vi "MK210.vi"(4 "error in":T13, 7 "Command":T14) -> (0 "error out":T13, 3 "Response":T11)   [LabVIEW 2018]
uses:
  MOKO_LabViewLibrary/MokoLowLevel/MokoLowLovelControl/MLLC_Command.ctl
  MOKO_LabViewLibrary/MokoLowLevel/MokoLowLovelControl/MLLC_Error.ctl
  MOKO_LabViewLibrary/MokoLowLevel/MokoLowLovelControl/MLLC_Mode.ctl
  MOKO_LabViewLibrary/MokoLowLevel/MokoLowLovelControl/MLLC_Response.ctl
  MOKO_LabViewLibrary/MokoLowLevel/MokoLowLovelControl/MLLC_DriverName.ctl
  MOKO_LabViewLibrary/MokoLowLevel/MokoLowLovelControl/MLLC_ResponseInit.ctl
  MOKO_LabViewLibrary/MokoLowLevel/MokoLowLovelControl/MLLC_Request.ctl
  MOKO_LabViewLibrary/MokoLowLevel/MokoLowLovelControl/MLLC_ErrorCode.ctl
  MOKO_LabViewLibrary/MokoLowLevel/MokoLowLovelControl/MLLC_ConnectCluster.ctl
  MOKO_LabViewLibrary/MokoLowLevel/MokoLowLovelControl/MLLC_InterfaceType.ctl
  MOKO_LabViewLibrary/MokoLowLevel/MokoLowLovelControl/MLLC_OpenedSession.ctl
  MOKO_LabViewLibrary/MokoLowLevel/MokoLowLovelControl/MLLC_InterfaceSettings.ctl
  MOKO_LabViewLibrary/MokoLowLevel/MokoLowLovelControl/MLLC_InterfaceKind.ctl
  MOKO_LabViewLibrary/MokoLowLevel/MokoLowLovelControl/MLLC_Rs232Settings.ctl
panel:
  in  "Settings":T6={"Permanent data"={"Connect"={"InterfaceType"=enum."VISA", "OpenedSession"="COM4", "InterfaceSettings"={"Interface"=enum."RS232", "EOS 4 read"=enum."Default (=EOS 4 write)", "EOS 4 write"=enum."CR (\\r)", "TMO, ms"=500, "Sett"=variant(cluster{"Baud Rate":u32, "Data Bits":u16, "Parity":u16, "Stop Bits":u16, "Flow Control":u16, "Eho":bool} {"Baud Rate"=75, "Data Bits"=0, "Parity"=0, "Stop Bits"=0, "Flow Control"=0, "Eho"=FALSE})}}}, "Saved Data"=variant}
  in  "Error Code":T7=5420
  in  "Request":T8="?MOD"
  in  "ResponseInit":T9="XP2I"
  in  "Driver Name":T10="MK210-301"
  in  "Mode":T12=enum."Check"
  # "MK210-301"
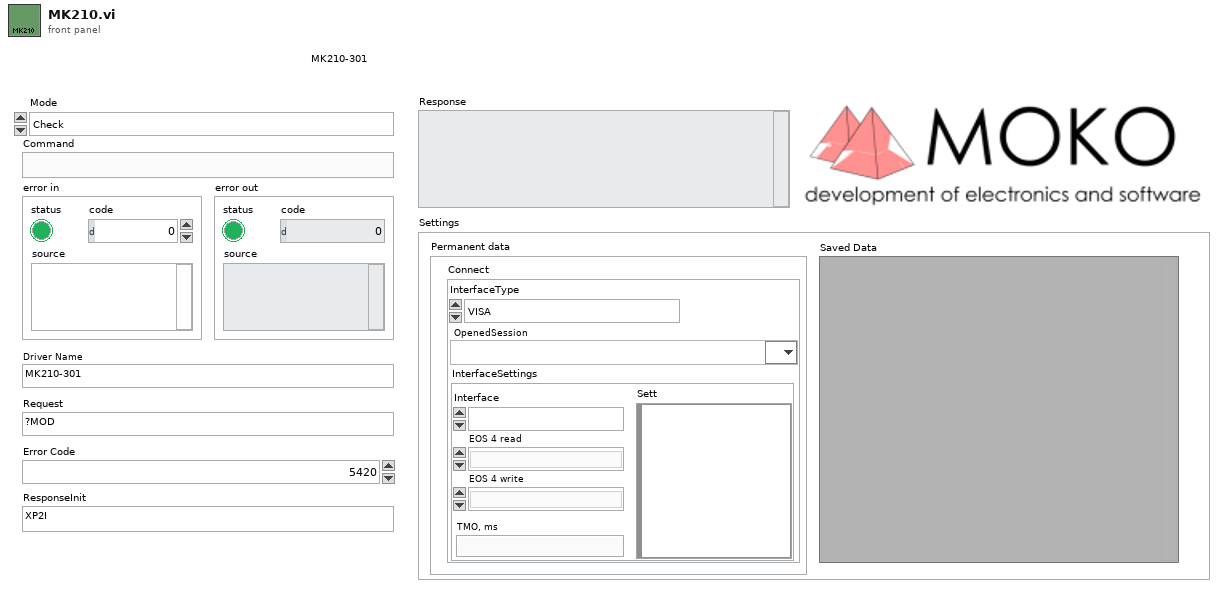
[diagram p1: front panel]
types:
  T1 = typedef "MLLC_ConnectCluster.ctl" = cluster{"InterfaceType":T2, "OpenedSession":T3, "InterfaceSettings":T4}
  T2 = typedef "MLLC_InterfaceType.ctl" = enum16{"VISA", "Prologix USB-GPIB"}
  T3 = typedef "MLLC_OpenedSession.ctl" = refnum<visa-resource-name>
  T4 = typedef "MLLC_InterfaceSettings.ctl" = cluster{"Interface":T5, "EOS 4 read":enum16{"Default (=EOS 4 write)", "CR (\\r)", "LF (\\n)", "None"}, "EOS 4 write":enum16{"CR+LF (\\r\\n)", "CR (\\r)", "LF (\\n)", "None"}, "TMO, ms":i32, "Sett":variant}
  T5 = typedef "MLLC_InterfaceKind.ctl" = enum16{"RS232", "GPIB", "USB", "Ethernet", "another"}
  T6 = cluster{"Permanent data":cluster{"Connect":T1}, "Saved Data":variant}
  T7 = typedef "MLLC_ErrorCode.ctl" = u32
  T8 = typedef "MLLC_Request.ctl" = string
  T9 = typedef "MLLC_ResponseInit.ctl" = string
  T10 = typedef "MLLC_DriverName.ctl" = string
  T11 = typedef "MLLC_Response.ctl" = string
  T12 = typedef "MLLC_Mode.ctl" = enum16{"get", "set", "close", "Init", "Check"}
  T13 = typedef "MLLC_Error.ctl" = errorcluster
  T14 = typedef "MLLC_Command.ctl" = string
  T15 = typedef "MLLC_Rs232Settings.ctl" = cluster{"Baud Rate":u32, "Data Bits":u16, "Parity":u16, "Stop Bits":u16, "Flow Control":u16, "Eho":bool, "Address":dbl}
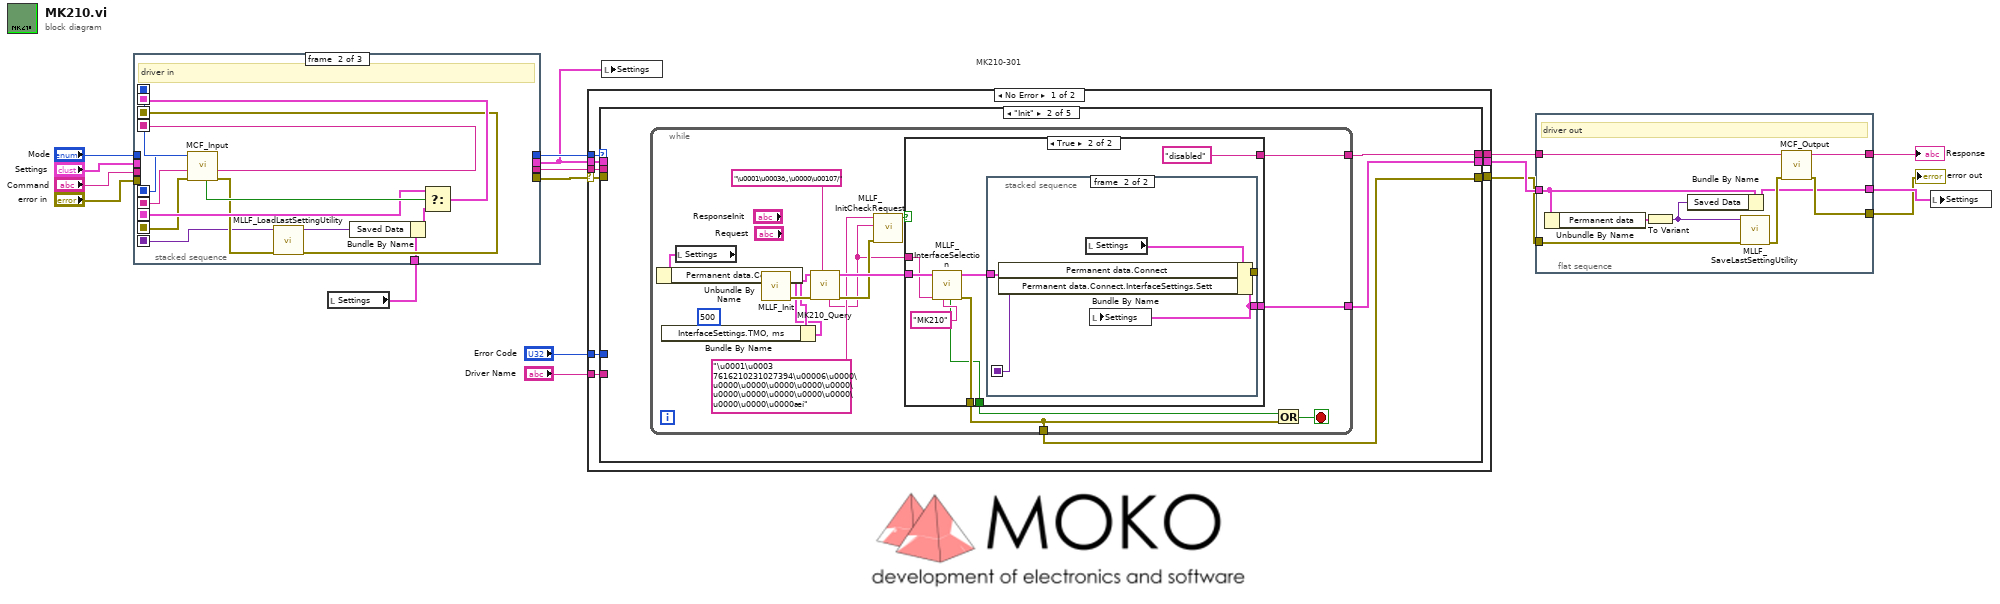
[diagram p0: block diagram]
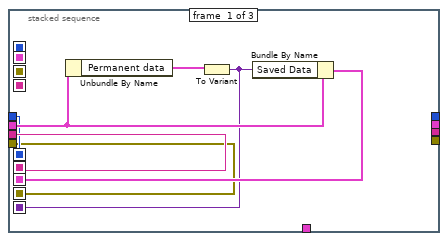
[diagram p2: hidden frame]
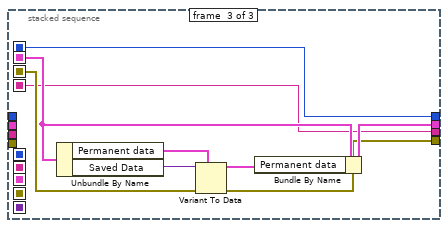
[diagram p3: hidden frame]
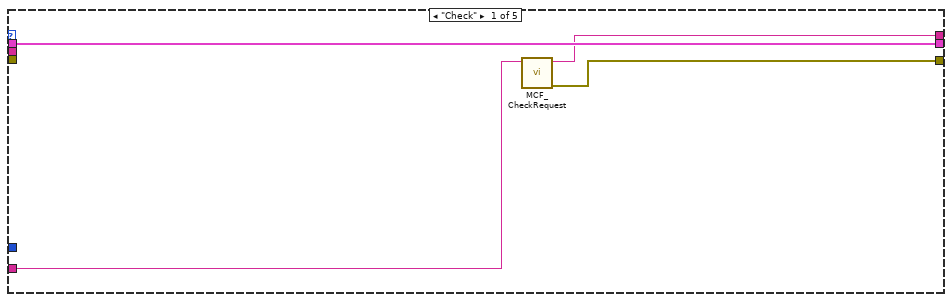
[diagram p4: hidden frame]
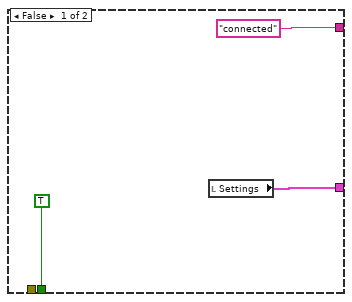
[diagram p5: hidden frame]
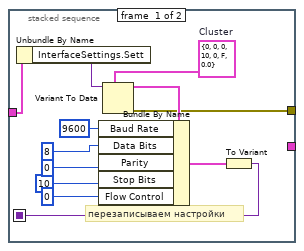
[diagram p6: hidden frame]
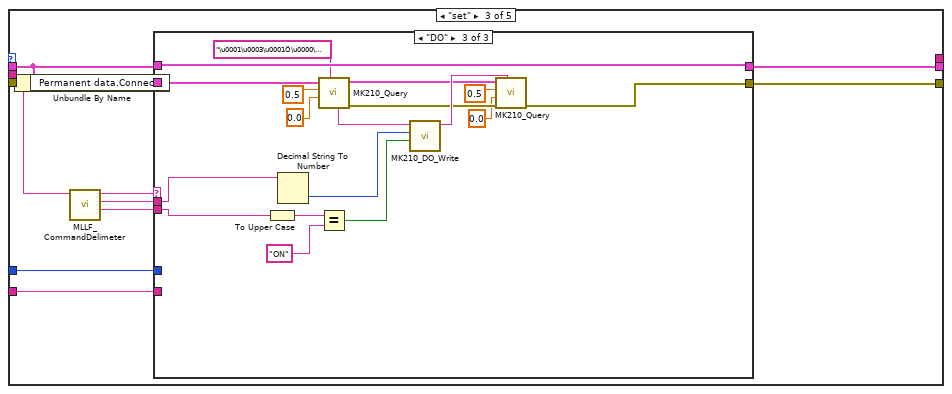
[diagram p7: hidden frame]
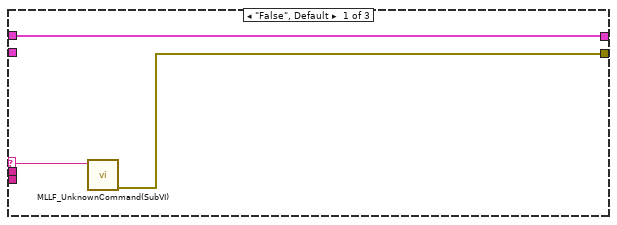
[diagram p8: hidden frame]
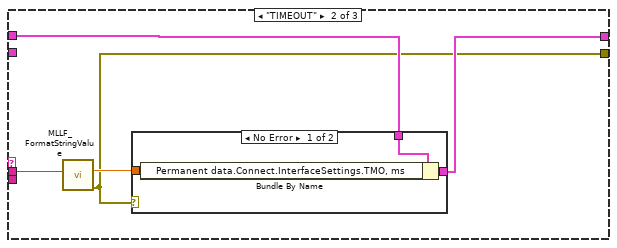
[diagram p9: hidden frame]
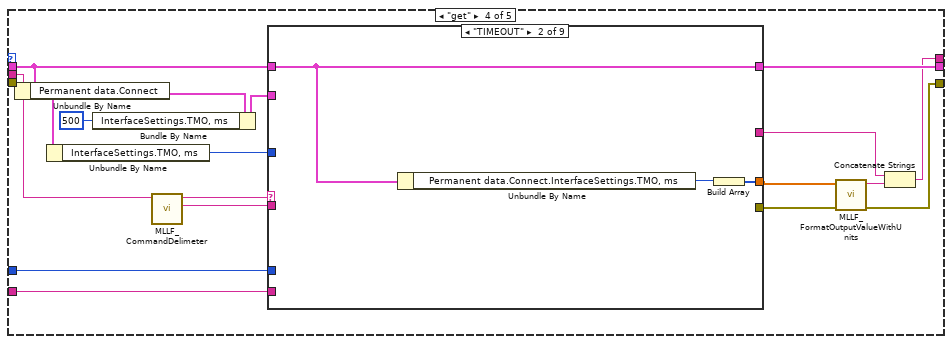
[diagram p11: hidden frame]
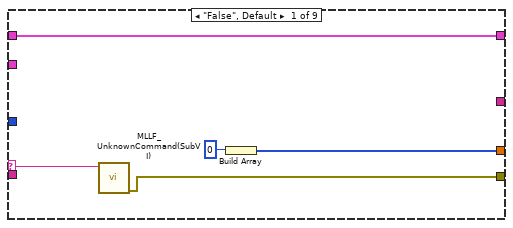
[diagram p12: hidden frame]
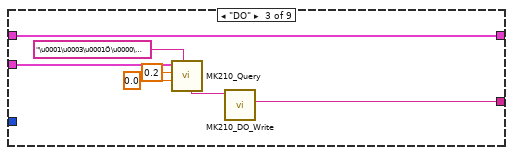
[diagram p13: hidden frame]
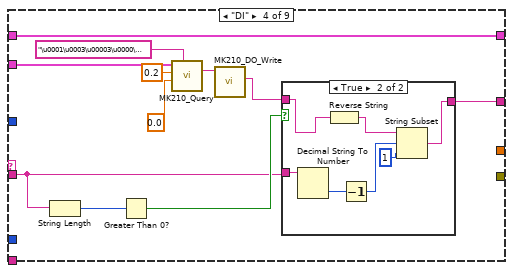
[diagram p14: hidden frame]
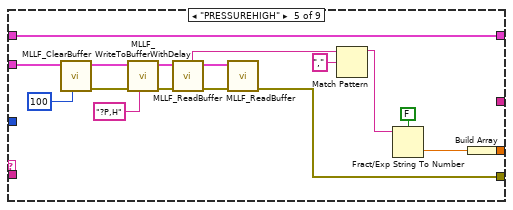
[diagram p16: hidden frame]
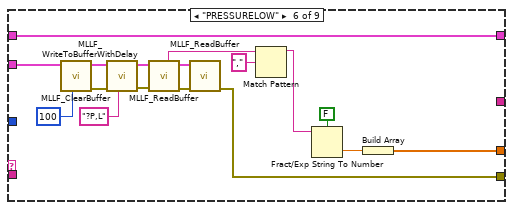
[diagram p17: hidden frame]
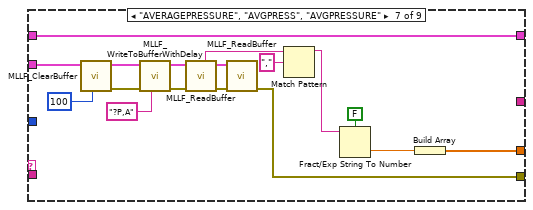
[diagram p18: hidden frame]
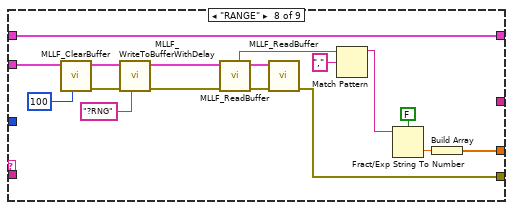
[diagram p19: hidden frame]
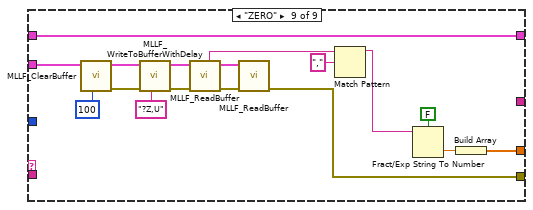
[diagram p20: hidden frame]
diagram:
  # "MK210-301"
  n1 = local read "Settings"() -> (w7:T6)
  n2 = stacked-sequence {
    seq-local: [w20 _ _] -> [_ w36 _]
    seq-local: [w19 _ _] -> [_ w37 _]
    seq-local: [w22 _ _] -> [_ w32 _]
    seq-local: [w18 _ _] -> [_ w31 _]
    seq-local: [w21 _ _] -> [_ w27 _]
    seq-local: [_ w28 _] -> [_ _ w44]
    seq-local: [_ w38 _] -> [_ _ w41]
    seq-local: [_ w35 _] -> [_ _ w40]
    seq-local: [_ w34 _] -> [_ _ w45]
    tunnel: "Command" -> [w20 _ _]
    tunnel: "Mode" -> [w19 _ _]
    tunnel: "error in" -> [w18 _ _]
    tunnel: "Settings" -> [w23 _ _]
    tunnel: w7 -> [_ w26 _]
    tunnel: [_ _ w40] -> w9
    tunnel: [_ _ w43] -> w10
    tunnel: [_ _ w42] -> w8
    tunnel: [_ _ w41] -> w11
    frame #0 {
      n3 = Unbundle By Name(w23) -> ("Permanent data"=w24:cluster{"Connect":T1})
      n4 = To Variant(anything=w24) -> (Variant=w21:variant)
      n5 = Bundle By Name(cluster=w23, "Saved Data"=w21) -> (w22:T6)
    }
    frame #1 {
      # "driver in"
      n6 = call "MCF_Input.vi"("Error In"=w31, "Command in"=w36, "Mode in"=w37) -> ("Error Out"=w30:errorcluster, "Command out"=w35:string, "Mode out"=w38:T12, "Boolean"=w33:bool)  [unwired: 5 in]
      n7 = call "MLLF_LoadLastSettingUtility.vi"("Error In"=w30, "Save data in"=w27) -> ("Error Out"=w28:errorcluster, "Save data out"=w25:variant)  [unwired: 8 in]
      n8 = Bundle By Name(cluster=w26, "Saved Data"=w25) -> (w29:T6)
      n9 = Select(t=w32, s=w33, f=w29) -> (s? t:f=w34:T6)
    }
    frame #2 {
      n10 = Unbundle By Name(w45) -> ("Permanent data"=w46:cluster{"Connect":T1}, "Saved Data"=w39:variant)
      n11 = Variant To Data(error in=w44, type=w46, Variant=w39) -> (data=w47:cluster{"Connect":T1}, error out=w42:errorcluster)
      n12 = Bundle By Name(cluster=w45, "Permanent data"=w47) -> (w43:T6)
    }
  }
  n13 = case shown="No Error" w8 {
    selector: w8 -> [w53 w289]
    tunnel: [w48 w289] -> w4
    tunnel: w11 -> [w56 _]
    tunnel: [w55 _] -> w6
    tunnel: w9 -> [w54 _]
    tunnel: w10 -> [w50 w288]
    tunnel: "Error Code" -> [w52 _]
    tunnel: "Driver Name" -> [w51 _]
    tunnel: [w49 w288] -> w5
    frame No Error {
      n14 = case shown="\"Init\"" w56 {
        tunnel: [w58 w63 _ w149 "" ("Output String")] -> w55
        tunnel: w54 -> [_ _ w112 w153 _]
        tunnel: w53 -> [_ _ _ _ _]
        tunnel: w52 -> [_ _ w117 w163 _]
        tunnel: w51 -> [w59 _ w114 w162 _]
        tunnel: w50 -> [w60 _ w116 w164 w286]
        tunnel: [w60 w62 w115 w161 w286] -> w49
        tunnel: [w57 w61 w109 w148 w285] -> w48
        frame "Check" {
          n15 = call "MCF_CheckRequest.vi"("Driver Name"=w59) -> ("Error Out"=w57:errorcluster, "Output String"=w58:string)  [unwired: 9 in]
        }
        frame "Init" {
          n16 = while {
            tunnel: [w78] -> w61
            tunnel: [w77] -> w63
            tunnel: [w76] -> w62
            stop <- w80 stop-if-true
            n17 = local read "Settings"() -> (w74:T6)
            n18 = Unbundle By Name(w74) -> ("Permanent data.Connect"=w73:T1)
            n19 = call "MLLF_Init.vi"("DriverConnect in"=w73) -> ("Error Out"=w72:errorcluster, "DriverConnect out"=w67:T1)  [unwired: 7 in]
            n20 = Bundle By Name(cluster=w67, "InterfaceSettings.TMO, ms"=500) -> (w65:T1)
            n21 = call "MK210_Query.vi"("String"="\u0001\u0003ð„\u0000\u00107/", "error in (no error)"=w72, "DriverConnect in"=w65) -> ("error out"=w70:errorcluster, "DriverConnect out"=w71:T1, "String from device out"=w64:string)  [unwired: 6 in]
            n22 = call "MLLF_InitCheckRequest.vi"("error in (no error)"=w70, "Answer"=w64, "Response Init"="\u0001\u0003 7616210231027394\u00006\u0000\u0000\u0000\u0000\u0000\u0000\u0000\u0000\u0000\u0000\u0000\u0000\u0000\u0000æí") -> ("Design"=w75:bool)  [unwired: 5 in, 3 out]
            n23 = case shown="True" w75 {
              tunnel: w71 -> [_ w90]
              tunnel: [TRUE w86] -> w79
              tunnel: [_ w91] -> w78
              tunnel: ["connected" "disabled"] -> w77
              tunnel: [w81 w85] -> w76
              tunnel: w64 -> [_ w84]
              frame False {
                n24 = local read "Settings"() -> (w81:T6)
              }
              frame True {
                n25 = call "MLLF_InterfaceSelection.vi"("Driver Name"="MK210" ("String"), "Answer:"=w84, "DriverConnect in"=w90) -> ("error out"=w91:T13, "DriverConnect out"=w89:T1, "stop init?"=w86:bool)  [unwired: 4 in, 2 out]
                n26 = stacked-sequence {
                  seq-local: [w95 _] -> [_ w104]
                  tunnel: w89 -> [w93 w105]
                  tunnel: [w96 _] -> _
                  tunnel: [_ w106] -> w85
                  frame #0 {
                    w97 = T15 {"Baud Rate"=0, "Data Bits"=0, "Parity"=0, "Stop Bits"=10, "Flow Control"=0, "Eho"=FALSE, "Address"=0.0}  # Cluster
                    # "перезаписываем настройки"
                    n27 = Unbundle By Name(w93) -> ("InterfaceSettings.Sett"=w92:variant)
                    n28 = Variant To Data(type=w97, Variant=w92) -> (data=w98:T15, error out=w96:errorcluster)  [unwired: 1 in]
                    n29 = Bundle By Name(cluster=w98, "Baud Rate"=u32 9600, "Data Bits"=u16 8 ("Serial Settings:Data Bits"), "Parity"=u16 0 ("Serial Settings:Parity"), "Stop Bits"=u16 10 ("Serial Settings:Stop Bits"), "Flow Control"=u16 0 ("Serial Settings:Flow Control")) -> (w103:T15)
                    n30 = To Variant(anything=w103) -> (Variant=w95:variant)
                  }
                  frame #1 {
                    n31 = local read "Settings"() -> (w107:T6)
                    n32 = Bundle By Name(cluster=w107, "Permanent data.Connect"=w105, "Permanent data.Connect.InterfaceSettings.Sett"=w104) -> (w106:T6)
                    n33 = local write "Settings"(w106) -> ()
                  }
                }
              }
            }
            n34 = Or(x=w79, y=w78) -> (x .or. y?=w80:bool)
          }
        }
        frame "set" {
          n35 = Unbundle By Name(w116) -> ("Permanent data.Connect"=w113:T1)
          n36 = call "MLLF_CommandDelimeter.vi"("command with param"=w112) -> ("param 2"=w108:string, "param 1"=w110:string, "command"=w111:string)  [unwired: 6 in, 2 out]
          n37 = case shown="\"DO\"" w111 {
            selector: w111 -> [w119 _ _]
            tunnel: w110 -> [_ w123 w131]
            tunnel: w117 -> [_ _ _]
            tunnel: w116 -> [w120 w124 w147]
            tunnel: [w120 w125 w147] -> w115
            tunnel: w114 -> [_ _ _]
            tunnel: [w118 w121 w143] -> w109
            tunnel: w113 -> [_ _ w137]
            tunnel: w108 -> [_ _ w130]
            frame "False", Default {
              n38 = call "MLLF_UnknownCommand(SubVI).vi"("Unknown command"=w119) -> ("error out"=w118:errorcluster)  [unwired: 10 in]
            }
            frame "TIMEOUT" {
              n39 = call "MLLF_FormatStringValue.vi"("String Value"=w123) -> ("error out"=w121:T13, "number"=w122:dbl)  [unwired: 8 in, 1 out]
              n40 = case shown="No Error" w121 {
                tunnel: [w128 w129] -> w125
                tunnel: w124 -> [w127 w129]
                tunnel: w122 -> [w126 _]
                frame No Error {
                  n41 = Bundle By Name(cluster=w127, "Permanent data.Connect.InterfaceSettings.TMO, ms"=w126) -> (w128:T6)
                }
                frame Error {
                }
              }
            }
            frame "DO" {
              n42 = To Upper Case(1:w130) -> (0:w141:string)
              n43 = Decimal String To Number(string=w131) -> (number=w139:i32)  [unwired: 2 in, 1 out]
              n44 = call "MK210_Query.vi"("String"="\u0001\u0003\u0001Ö\u0000\u0001d\u000e", "Delay Time (s) 2"=0.0, "Delay Time (s)"=0.5, "DriverConnect in"=w137) -> ("error out"=w136:errorcluster, "DriverConnect out"=w138:T1, "String from device out"=w145:string)  [unwired: 5 in]
              n45 = Equal?(x=w141, y="ON") -> (x = y?=w140:bool)
              n46 = call "MK210_DO_Write.vi"("Button"=w140, "n of on"=w139, "Sustain"=w145) -> ("concatenated string"=w144:string)  [unwired: 6 in, 2 out]
              n47 = call "MK210_Query.vi"("String"=w144, "error in (no error)"=w136, "Delay Time (s) 2"=0.0, "Delay Time (s)"=0.5, "DriverConnect in"=w138) -> ("error out"=w143:errorcluster)  [unwired: 4 in, 2 out]
            }
          }
        }
        frame "get" {
          n48 = Unbundle By Name(w164) -> ("Permanent data.Connect"=w150:T1)
          n49 = Unbundle By Name(w150) -> ("InterfaceSettings.TMO, ms"=w158:i32)
          n50 = Bundle By Name(cluster=w150, "InterfaceSettings.TMO, ms"=500) -> (w154:T1)
          n51 = call "MLLF_CommandDelimeter.vi"("command with param"=w153) -> ("param 1"=w151:string, "command"=w152:string)  [unwired: 6 in, 3 out]
          n52 = case shown="\"TIMEOUT\"" w152 {
            selector: w152 -> [w166 _ _ _ _ _ _ _ _]
            tunnel: w151 -> [_ _ _ w180 _ _ _ _ _]
            tunnel: [w165 _ _ _ w208 w225 w242 w259 w276] -> w160
            tunnel: w163 -> [_ _ _ _ _ _ _ _ _]
            tunnel: [w169 w172 w179 w190 w215 w232 w249 w266 w283] -> w161
            tunnel: w164 -> [w169 w172 w179 w190 w215 w232 w249 w266 w283]
            tunnel: [w167 w170 _ _ w212 w229 w246 w263 w280] -> w159
            tunnel: w162 -> [_ _ _ _ _ _ _ _ _]
            tunnel: w158 -> [_ _ _ _ _ _ _ _ _]
            tunnel: [_ _ w175 w183 _ _ _ _ _] -> w156
            tunnel: w154 -> [_ _ w176 w187 w199 w216 w233 w250 w267]
            frame "False", Default {
              n53 = call "MLLF_UnknownCommand(SubVI).vi"("Unknown command"=w166) -> ("error out"=w165:errorcluster)  [unwired: 10 in]
              n54 = Build Array(0 ("TimeOut")) -> (w167:i32[])
            }
            frame "TIMEOUT" {
              n55 = Unbundle By Name(w172) -> ("Permanent data.Connect.InterfaceSettings.TMO, ms"=w171:i32)
              n56 = Build Array(w171) -> (w170:i32[])
            }
            frame "DO" {
              n57 = call "MK210_Query.vi"("String"="\u0001\u0003\u0001Ö\u0000\u0001d\u000e", "Delay Time (s) 2"=0.0, "Delay Time (s)"=0.2, "DriverConnect in"=w176) -> ("String from device out"=w177:string)  [unwired: 5 in, 2 out]
              n58 = call "MK210_DO_Write.vi"("Sustain"=w177) -> ("BIN OUT"=w175:string)  [unwired: 8 in, 2 out]
            }
            frame "DI" {
              n59 = String Length(string=w180) -> (length=w186:i32)
              n60 = Greater Than 0?(x=w186) -> (x > 0?=w185:bool)
              n61 = call "MK210_Query.vi"("String"="\u0001\u0003\u00003\u0000\u0001t\u0005", "Delay Time (s) 2"=0.0, "Delay Time (s)"=0.2, "DriverConnect in"=w187) -> ("String from device out"=w188:string)  [unwired: 5 in, 2 out]
              n62 = call "MK210_DO_Write.vi"("Sustain"=w188) -> ("BIN OUT"=w184:string)  [unwired: 8 in, 2 out]
              n63 = case shown="True" w185 {
                tunnel: w184 -> [w191 w193]
                tunnel: [w191 w197] -> w183
                tunnel: w180 -> [_ w198]
                frame False {
                }
                frame True {
                  n64 = Decimal String To Number(string=w198) -> (number=w196:i32)  [unwired: 2 in, 1 out]
                  n65 = Reverse String(1:w193) -> (0:w192:string)
                  n66 = Decrement(x=w196) -> (x-1=w195:i32)
                  n67 = String Subset(string=w192, offset (0)=w195, length (rest)=1 ("length (rest)")) -> (substring=w197:string)
                }
              }
            }
            frame "PRESSUREHIGH" {
              n68 = call "MLLF_ClearBuffer.vi"("Timeout(default = 300 ms)"=u32 100 ("Timeout"), "DriverConnect in"=w199) -> ("Error Out"=w209:errorcluster, "DriverConnect out"=w210:T1)  [unwired: 6 in, 1 out]
              n69 = call "MLLF_WriteToBufferWithDelay.vi"("Command"="?P,H" ("String"), "Error In"=w209, "DriverConnect in"=w210) -> ("Error Out"=w201:errorcluster, "DriverConnect out"=w205:T1)  [unwired: 7 in]
              n70 = call "MLLF_ReadBuffer.vi"("Error In"=w201, "DriverConnect in"=w205) -> ("Error Out"=w204:errorcluster, "DriverConnect out"=w203:T1, "String"=w202:string)  [unwired: 6 in]
              n71 = call "MLLF_ReadBuffer.vi"("Error In"=w204, "DriverConnect in"=w203) -> ("Error Out"=w208:errorcluster)  [unwired: 6 in, 2 out]
              n72 = Match Pattern(string=w202, regular expression=",") -> (before substring=w206:string)  [unwired: 1 in, 3 out]
              n73 = Fract/Exp String To Number(use system decimal point (T)=FALSE, string=w206) -> (number=w213:dbl)  [unwired: 2 in, 1 out]
              n74 = Build Array(w213) -> (w212:dbl[])
            }
            frame "PRESSURELOW" {
              n75 = call "MLLF_ClearBuffer.vi"("Timeout(default = 300 ms)"=u32 100 ("Timeout"), "DriverConnect in"=w216) -> ("Error Out"=w226:errorcluster, "DriverConnect out"=w227:T1)  [unwired: 6 in, 1 out]
              n76 = call "MLLF_WriteToBufferWithDelay.vi"("Command"="?P,L" ("String"), "Error In"=w226, "DriverConnect in"=w227) -> ("Error Out"=w218:errorcluster, "DriverConnect out"=w222:T1)  [unwired: 7 in]
              n77 = call "MLLF_ReadBuffer.vi"("Error In"=w218, "DriverConnect in"=w222) -> ("Error Out"=w221:errorcluster, "DriverConnect out"=w220:T1, "String"=w219:string)  [unwired: 6 in]
              n78 = call "MLLF_ReadBuffer.vi"("Error In"=w221, "DriverConnect in"=w220) -> ("Error Out"=w225:errorcluster)  [unwired: 6 in, 2 out]
              n79 = Match Pattern(string=w219, regular expression=",") -> (before substring=w223:string)  [unwired: 1 in, 3 out]
              n80 = Fract/Exp String To Number(use system decimal point (T)=FALSE, string=w223) -> (number=w230:dbl)  [unwired: 2 in, 1 out]
              n81 = Build Array(w230) -> (w229:dbl[])
            }
            frame "AVERAGEPRESSURE", "AVGPRESS", "AVGPRESSURE" {
              n82 = call "MLLF_ClearBuffer.vi"("Timeout(default = 300 ms)"=u32 100 ("Timeout"), "DriverConnect in"=w233) -> ("Error Out"=w243:errorcluster, "DriverConnect out"=w244:T1)  [unwired: 6 in, 1 out]
              n83 = call "MLLF_WriteToBufferWithDelay.vi"("Command"="?P,A" ("String"), "Error In"=w243, "DriverConnect in"=w244) -> ("Error Out"=w235:errorcluster, "DriverConnect out"=w239:T1)  [unwired: 7 in]
              n84 = call "MLLF_ReadBuffer.vi"("Error In"=w235, "DriverConnect in"=w239) -> ("Error Out"=w238:errorcluster, "DriverConnect out"=w237:T1, "String"=w236:string)  [unwired: 6 in]
              n85 = call "MLLF_ReadBuffer.vi"("Error In"=w238, "DriverConnect in"=w237) -> ("Error Out"=w242:errorcluster)  [unwired: 6 in, 2 out]
              n86 = Match Pattern(string=w236, regular expression=",") -> (before substring=w240:string)  [unwired: 1 in, 3 out]
              n87 = Fract/Exp String To Number(use system decimal point (T)=FALSE, string=w240) -> (number=w247:dbl)  [unwired: 2 in, 1 out]
              n88 = Build Array(w247) -> (w246:dbl[])
            }
            frame "RANGE" {
              n89 = call "MLLF_ClearBuffer.vi"("Timeout(default = 300 ms)"=u32 100 ("Timeout"), "DriverConnect in"=w250) -> ("Error Out"=w260:errorcluster, "DriverConnect out"=w261:T1)  [unwired: 6 in, 1 out]
              n90 = call "MLLF_WriteToBufferWithDelay.vi"("Command"="?RNG" ("String"), "Error In"=w260, "DriverConnect in"=w261) -> ("Error Out"=w252:errorcluster, "DriverConnect out"=w256:T1)  [unwired: 7 in]
              n91 = call "MLLF_ReadBuffer.vi"("Error In"=w252, "DriverConnect in"=w256) -> ("Error Out"=w255:errorcluster, "DriverConnect out"=w254:T1, "String"=w253:string)  [unwired: 6 in]
              n92 = call "MLLF_ReadBuffer.vi"("Error In"=w255, "DriverConnect in"=w254) -> ("Error Out"=w259:errorcluster)  [unwired: 6 in, 2 out]
              n93 = Match Pattern(string=w253, regular expression=",") -> (before substring=w257:string)  [unwired: 1 in, 3 out]
              n94 = Fract/Exp String To Number(use system decimal point (T)=FALSE, string=w257) -> (number=w264:dbl)  [unwired: 2 in, 1 out]
              n95 = Build Array(w264) -> (w263:dbl[])
            }
            frame "ZERO" {
              n96 = call "MLLF_ClearBuffer.vi"("Timeout(default = 300 ms)"=u32 100 ("Timeout"), "DriverConnect in"=w267) -> ("Error Out"=w277:errorcluster, "DriverConnect out"=w278:T1)  [unwired: 6 in, 1 out]
              n97 = call "MLLF_WriteToBufferWithDelay.vi"("Command"="?Z,U" ("String"), "Error In"=w277, "DriverConnect in"=w278) -> ("Error Out"=w269:errorcluster, "DriverConnect out"=w273:T1)  [unwired: 7 in]
              n98 = call "MLLF_ReadBuffer.vi"("Error In"=w269, "DriverConnect in"=w273) -> ("Error Out"=w272:errorcluster, "DriverConnect out"=w271:T1, "String"=w270:string)  [unwired: 6 in]
              n99 = call "MLLF_ReadBuffer.vi"("Error In"=w272, "DriverConnect in"=w271) -> ("Error Out"=w276:errorcluster)  [unwired: 6 in, 2 out]
              n100 = Match Pattern(string=w270, regular expression=",") -> (before substring=w274:string)  [unwired: 1 in, 3 out]
              n101 = Fract/Exp String To Number(use system decimal point (T)=FALSE, string=w274) -> (number=w281:dbl)  [unwired: 2 in, 1 out]
              n102 = Build Array(w281) -> (w280:dbl[])
            }
          }
          n103 = call "MLLF_FormatOutputValueWithUnits.vi"("error in"=w160, "ValuesIn"=w159) -> ("error out"=w148:T13, "Result string"=w157:T14)  [unwired: 8 in]
          n104 = Concatenate Strings(w156, w157) -> (w149:string)
        }
        frame "close" {
          n105 = Unbundle By Name(w286) -> ("Permanent data.Connect.OpenedSession"=w287:T3)
          n106 = VISA Close(VISA resource name=w287) -> (error out=w285:errorcluster)  [unwired: 1 in]
        }
      }
    }
    frame Error {
    }
  }
  n107 = local write "Settings"(w10) -> ()
  n108 = flat-sequence {
    tunnel: [w298] -> w3
    tunnel: [w297] -> w1
    tunnel: w6 -> [w296]
    tunnel: w4 -> [w295]
    tunnel: w5 -> [w291]
    tunnel: [w293] -> w2
    frame #0 {
      # "driver out"
      n109 = Unbundle By Name(w291) -> ("Permanent data"=w290:cluster{"Connect":T1})
      n110 = To Variant(anything=w290) -> (Variant=w292:variant)
      n111 = Bundle By Name(cluster=w291, "Saved Data"=w292) -> (w293:T6)
      n112 = call "MLLF_SaveLastSettingUtility.vi"("error in"=w295, "Saved Data"=w292) -> ("error out"=w294:T13)  [unwired: 8 in, 1 out]
      n113 = call "MCF_Output.vi"("Error In"=w294, "Input"=w296) -> ("Error Out"=w297:errorcluster, "Output"=w298:string)  [unwired: 8 in]
    }
  }
  n114 = local write "Settings"(w2) -> ()
  "error out" <- w1
  "Response" <- w3
